vi "session_set_one_property_boolean.vi"(6 "Skip setting if in Options string (F)":bool, 7 "Session Parameter Boolean":T1, 8 "error in":errorcluster caption="error in (no error)", 10 "Boolean value in":bool, 11 "VISA resource name":refnum<visa-resource-name>) -> (0 "error out":errorcluster, 2 "Set in the Options string":bool, 3 "VISA resource name out":refnum<visa-resource-name>)   [LabVIEW 2020, in "Rohde&Schwarz RTx Oscilloscopes.lvlib" / "rsidr_core.lvlib"]
uses:
  rsidr_core.lvlib
  type_Session_Parameter_Boolean.ctl
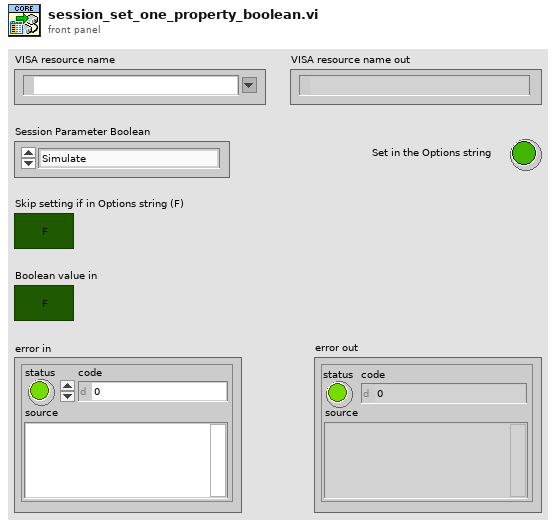
[diagram p1: front panel]
types:
  T1 = typedef "Rohde&Schwarz RTx Oscilloscopes.lvlib/rsidr_core.lvlib/type_Session_Parameter_Boolean.ctl" = enum16{"Simulate", "Query Instr Status", "Check Range", "Check Options", "Add LF to Write", "Duplicate Session", "Fast Sweep", "Logging", "OPC-sync Attribute Queries", "OPC-sync Attribute Writes"}
  T2 = typedef "Rohde&Schwarz RTx Oscilloscopes.lvlib/rsidr_core.lvlib/type_Session_Data.ctl" = cluster{"IDN string":string, "Instrument FW":string, "Instr type":string, "Instr type for err. msg.":string, "Installed Options":string[], "Ignore Error Messages":string, "Logging params":variant, "OPC Timeout":i32, "VISA Timeout":i32, "STB Poll VISA Timeout":i32, "Additional Flags":i32, "Wait Before Read":i32, "Wait Before Write":i32, "Option String Flags":i32, "IO Segment Size":i64, "VISA Access Mode":T3, "Interface Type":T4, "OPC Wait Mode":T5, "Bin Float Number  Format":T6, "Bin Integer Number Format":T7, "Simulate":bool, "VXIcapable":bool, "Duplicate Session":bool, "Add LF to Write":bool, "Logging":bool, "Fast Sweep":bool, "Query Instrument Status":bool, "Check Range":bool, "Check Options":bool, "OPC-sync Attr Writes":bool, "OPC-sync Attr Queries":bool}
  T3 = typedef "Rohde&Schwarz RTx Oscilloscopes.lvlib/rsidr_core.lvlib/type_VisaAccessMode.ctl" = u16
  T4 = typedef "Rohde&Schwarz RTx Oscilloscopes.lvlib/rsidr_core.lvlib/type_InterfaceType.ctl" = enum16{"Unknown", "GPIB", "VXI", "GPIB_VXI", "ASRL", "PXI", "TCPIP", "USB", "SOCKET"}
  T5 = typedef "Rohde&Schwarz RTx Oscilloscopes.lvlib/rsidr_core.lvlib/type_OPC_Wait_Mode.ctl" = enum16{"STBpolling", "STBpollingSlow", "STBpollingSuperSlow", "ServiceRequest", "OPCquery"}
  T6 = typedef "Rohde&Schwarz RTx Oscilloscopes.lvlib/rsidr_core.lvlib/type_Binary_Float_Number_Format.ctl" = enum16{"Float_4_Bytes_Swapped", "Float_4_Bytes", "Double_8_Bytes_Swapped", "Double_8_Bytes"}
  T7 = typedef "Rohde&Schwarz RTx Oscilloscopes.lvlib/rsidr_core.lvlib/type_Binary_Integer_Number_Format.ctl" = enum16{"Int32_4_Bytes_Swapped", "Int32_4 Bytes", "Int16_2_Bytes_Swapped", "Int16_2_Bytes"}
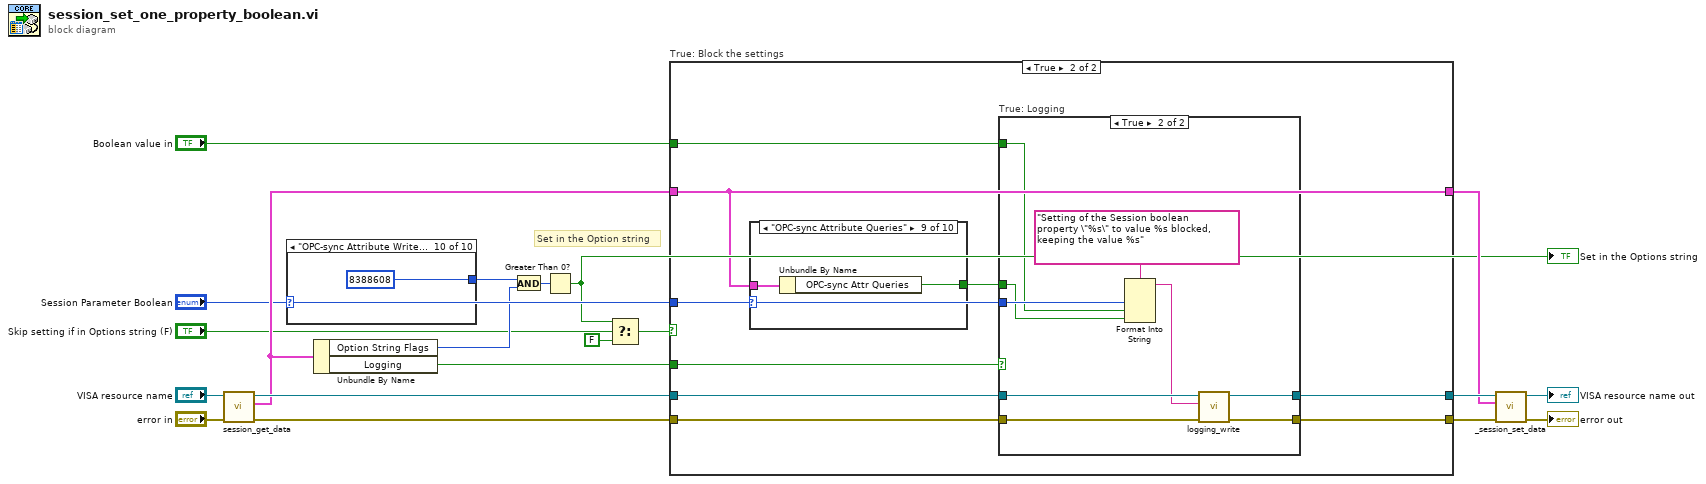
[diagram p0: block diagram]
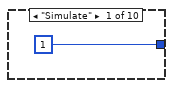
[diagram p2: hidden frame]
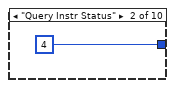
[diagram p3: hidden frame]
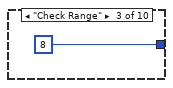
[diagram p4: hidden frame]
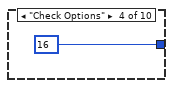
[diagram p5: hidden frame]
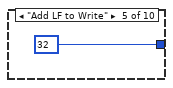
[diagram p6: hidden frame]
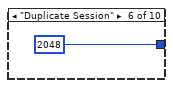
[diagram p7: hidden frame]
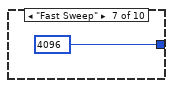
[diagram p8: hidden frame]
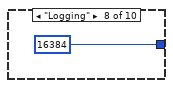
[diagram p9: hidden frame]
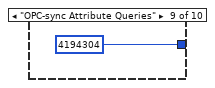
[diagram p10: hidden frame]
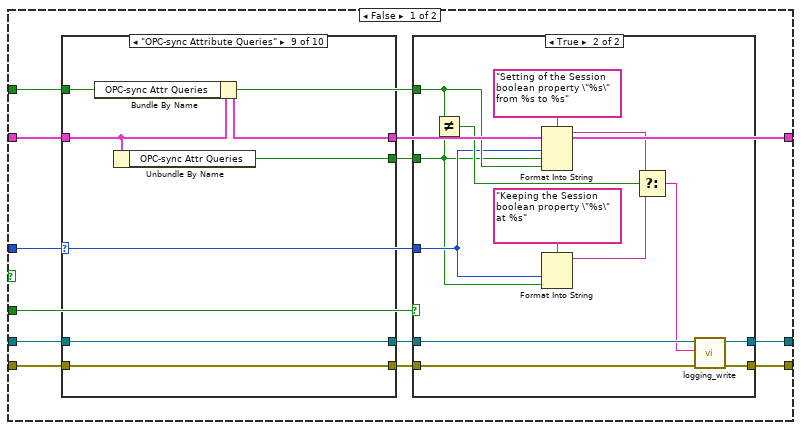
[diagram p11: hidden frame]
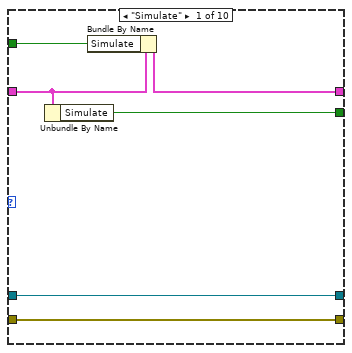
[diagram p13: hidden frame]
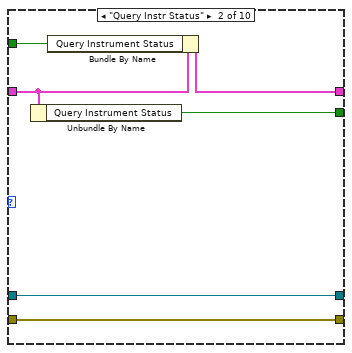
[diagram p14: hidden frame]
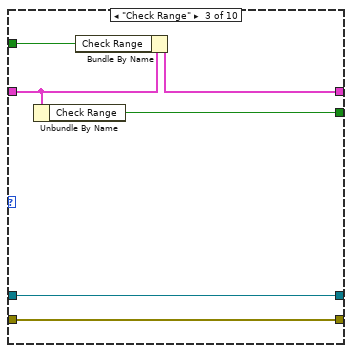
[diagram p15: hidden frame]
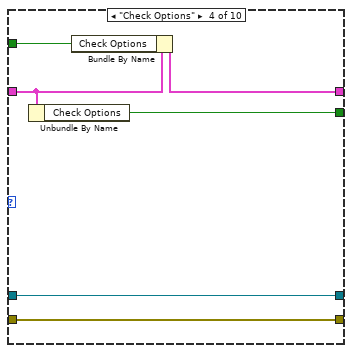
[diagram p16: hidden frame]
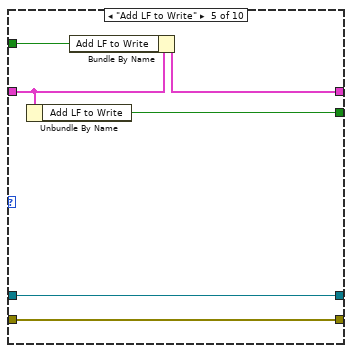
[diagram p17: hidden frame]
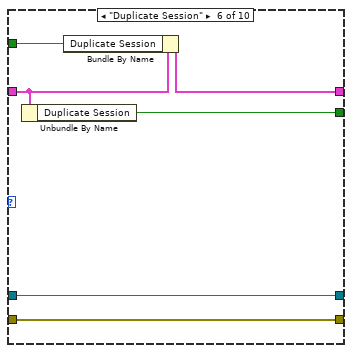
[diagram p18: hidden frame]
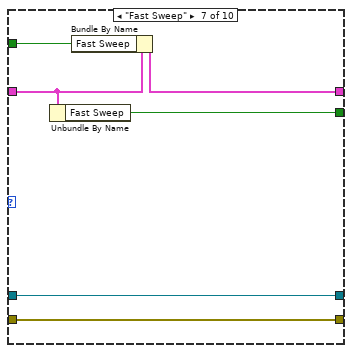
[diagram p19: hidden frame]
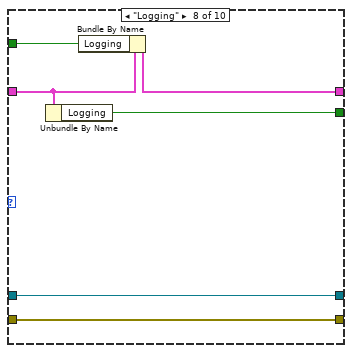
[diagram p20: hidden frame]
diagram:
  # "Set in the Option string"
  n1 = call "session_get_data.vi"("error in"="error in", "VISA resource name"="VISA resource name") -> ("error out"=w17:errorcluster, "Session User Data out"=w11:T2, "VISA resource name out"=w16:refnum<visa-resource-name>)  [unwired: 6 in, 1 out]
  n2 = case shown="\"OPC-sync Attribute Writes\"" "Session Parameter Boolean" {
    tunnel: [1 4 8 16 32 2048 4096 16384 4194304 8388608] -> w7
    frame "Simulate" {
    }
    frame "Query Instr Status" {
    }
    frame "Check Range" {
    }
    frame "Check Options" {
    }
    frame "Add LF to Write" {
    }
    frame "Duplicate Session" {
    }
    frame "Fast Sweep" {
    }
    frame "Logging" {
    }
    frame "OPC-sync Attribute Queries" {
    }
    frame "OPC-sync Attribute Writes" {
    }
  }
  n3 = Unbundle By Name(w11) -> ("Option String Flags"=w6:i32, "Logging"=w8:bool)
  n4 = And(x=w7, y=w6) -> (x .and. y?=w4:i32)
  n5 = Greater Than 0?(x=w4) -> (x > 0?=w2:bool)
  "Set in the Options string" <- w2
  n6 = Select(t=w2, s="Skip setting if in Options string (F)", f=FALSE) -> (s? t:f=w3:bool)
  n7 = case "True: Block the settings" shown="True" w3 {
    tunnel: "Session Parameter Boolean" -> [w35 w120]
    tunnel: w11 -> [w42 w119]
    tunnel: "Boolean value in" -> [w37 w121]
    tunnel: [w41 w119] -> w10
    tunnel: w17 -> [w40 w125]
    tunnel: w16 -> [w39 w124]
    tunnel: [w32 w123] -> w15
    tunnel: [w31 w122] -> w14
    tunnel: w8 -> [w36 w126]
    frame False {
      n8 = case shown="\"OPC-sync Attribute Queries\"" w35 {
        tunnel: w37 -> [w63 w69 w75 w81 w87 w93 w99 w105 w111 w117]
        tunnel: w42 -> [w59 w65 w71 w77 w83 w89 w95 w101 w107 w113]
        tunnel: [w60 w66 w72 w78 w84 w90 w96 w102 w108 w114] -> w41
        tunnel: w40 -> [w61 w68 w74 w80 w86 w92 w97 w103 w109 w115]
        tunnel: w39 -> [w62 w67 w73 w79 w85 w91 w98 w104 w110 w116]
        tunnel: [w61 w68 w74 w80 w86 w92 w97 w103 w109 w115] -> w34
        tunnel: [w62 w67 w73 w79 w85 w91 w98 w104 w110 w116] -> w33
        tunnel: [w58 w64 w70 w76 w82 w88 w94 w100 w106 w112] -> w38
        frame "Simulate" {
          n9 = Unbundle By Name(w59) -> ("Simulate"=w58:bool)
          n10 = Bundle By Name(cluster=w59, "Simulate"=w63) -> (w60:T2)
        }
        frame "Query Instr Status" {
          n11 = Unbundle By Name(w65) -> ("Query Instrument Status"=w64:bool)
          n12 = Bundle By Name(cluster=w65, "Query Instrument Status"=w69) -> (w66:T2)
        }
        frame "Check Range" {
          n13 = Unbundle By Name(w71) -> ("Check Range"=w70:bool)
          n14 = Bundle By Name(cluster=w71, "Check Range"=w75) -> (w72:T2)
        }
        frame "Check Options" {
          n15 = Unbundle By Name(w77) -> ("Check Options"=w76:bool)
          n16 = Bundle By Name(cluster=w77, "Check Options"=w81) -> (w78:T2)
        }
        frame "Add LF to Write" {
          n17 = Unbundle By Name(w83) -> ("Add LF to Write"=w82:bool)
          n18 = Bundle By Name(cluster=w83, "Add LF to Write"=w87) -> (w84:T2)
        }
        frame "Duplicate Session" {
          n19 = Unbundle By Name(w89) -> ("Duplicate Session"=w88:bool)
          n20 = Bundle By Name(cluster=w89, "Duplicate Session"=w93) -> (w90:T2)
        }
        frame "Fast Sweep" {
          n21 = Unbundle By Name(w95) -> ("Fast Sweep"=w94:bool)
          n22 = Bundle By Name(cluster=w95, "Fast Sweep"=w99) -> (w96:T2)
        }
        frame "Logging" {
          n23 = Unbundle By Name(w101) -> ("Logging"=w100:bool)
          n24 = Bundle By Name(cluster=w101, "Logging"=w105) -> (w102:T2)
        }
        frame "OPC-sync Attribute Queries" {
          n25 = Bundle By Name(cluster=w107, "OPC-sync Attr Queries"=w111) -> (w108:T2)
          n26 = Unbundle By Name(w107) -> ("OPC-sync Attr Queries"=w106:bool)
        }
        frame "OPC-sync Attribute Writes" {
          n27 = Bundle By Name(cluster=w113, "OPC-sync Attr Writes"=w117) -> (w114:T2)
          n28 = Unbundle By Name(w113) -> ("OPC-sync Attr Writes"=w112:bool)
        }
      }
      n29 = case shown="True" w36 {
        tunnel: w38 -> [_ w45]
        tunnel: w37 -> [_ w47]
        tunnel: w35 -> [_ w46]
        tunnel: w34 -> [w43 w53]
        tunnel: w33 -> [w44 w52]
        tunnel: [w43 w51] -> w32
        tunnel: [w44 w50] -> w31
        frame False {
        }
        frame True {
          n30 = Not Equal?(x=w47, y=w45) -> (x != y?=w48:bool)
          n31 = Format Into String(format string="Setting of the Session boolean property \"%s\" from %s to %s", w46, w45, w47) -> (resulting string=w56:string)  [unwired: 2 in, 1 out]
          n32 = Format Into String(format string="Keeping the Session boolean property \"%s\" at %s", w46, w45) -> (resulting string=w57:string)  [unwired: 2 in, 1 out]
          n33 = Select(t=w56, s=w48, f=w57) -> (s? t:f=w49:string)
          n34 = call "logging_write.vi"("error in"=w53, "String to write"=w49, "VISA resource name"=w52) -> ("error out"=w51:errorcluster, "VISA resource name out"=w50:refnum<visa-resource-name>)  [unwired: 7 in]
        }
      }
    }
    frame True {
      n35 = case shown="\"OPC-sync Attribute Queries\"" w120 {
        tunnel: w119 -> [w128 w130 w132 w134 w136 w138 w140 w142 w144 w146]
        tunnel: [w127 w129 w131 w133 w135 w137 w139 w141 w143 w145] -> w118
        frame "Simulate" {
          n36 = Unbundle By Name(w128) -> ("Simulate"=w127:bool)
        }
        frame "Query Instr Status" {
          n37 = Unbundle By Name(w130) -> ("Query Instrument Status"=w129:bool)
        }
        frame "Check Range" {
          n38 = Unbundle By Name(w132) -> ("Check Range"=w131:bool)
        }
        frame "Check Options" {
          n39 = Unbundle By Name(w134) -> ("Check Options"=w133:bool)
        }
        frame "Add LF to Write" {
          n40 = Unbundle By Name(w136) -> ("Add LF to Write"=w135:bool)
        }
        frame "Duplicate Session" {
          n41 = Unbundle By Name(w138) -> ("Duplicate Session"=w137:bool)
        }
        frame "Fast Sweep" {
          n42 = Unbundle By Name(w140) -> ("Fast Sweep"=w139:bool)
        }
        frame "Logging" {
          n43 = Unbundle By Name(w142) -> ("Logging"=w141:bool)
        }
        frame "OPC-sync Attribute Queries" {
          n44 = Unbundle By Name(w144) -> ("OPC-sync Attr Queries"=w143:bool)
        }
        frame "OPC-sync Attribute Writes" {
          n45 = Unbundle By Name(w146) -> ("OPC-sync Attr Writes"=w145:bool)
        }
      }
      n46 = case "True: Logging" shown="True" w126 {
        tunnel: w125 -> [w148 w157]
        tunnel: w124 -> [w147 w156]
        tunnel: [w148 w155] -> w123
        tunnel: [w147 w154] -> w122
        tunnel: w120 -> [_ w153]
        tunnel: w121 -> [_ w150]
        tunnel: w118 -> [_ w149]
        frame False {
        }
        frame True {
          n47 = Format Into String(format string="Setting of the Session boolean property \"%s\" to value %s blocked, keeping the value %s", w153, w150, w149) -> (resulting string=w151:string)  [unwired: 2 in, 1 out]
          n48 = call "logging_write.vi"("error in"=w157, "String to write"=w151, "VISA resource name"=w156) -> ("error out"=w155:errorcluster, "VISA resource name out"=w154:refnum<visa-resource-name>)  [unwired: 7 in]
        }
      }
    }
  }
  n49 = call "_session_set_data.vi"("error in"=w15, "Session User Data in"=w10, "VISA resource name"=w14) -> ("error out"=→"error out":errorcluster, "VISA resource name out"=→"VISA resource name out":refnum<visa-resource-name>)  [unwired: 7 in]
